vi "New Image.vi"(8 "error in (no error)":errorcluster, 9 "Buffer Number":i32, 10 "Image":T1, 11 "IMAQ Display in":refnum<class "HIJ Vision Display.lvclass">) -> (0 "error out":errorcluster, 3 "IMAQ Display out":refnum<class "HIJ Vision Display.lvclass">)   [LabVIEW 2014, in "HIJ Vision Display.lvlib" / "HIJ Vision Display.lvclass"]
uses:
  HIJ Vision Display.lvclass
  <vilib>/vision/Image Controls.llb/IMAQ Image.ctl
  HIJ Vision Display.lvclass/HIJ Vision Display.ctl
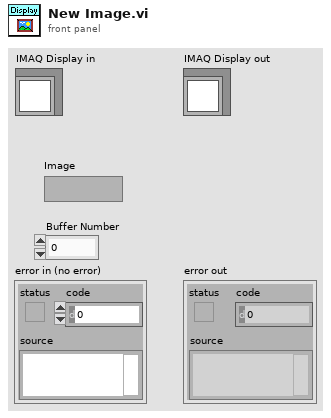
[diagram p1: front panel]
types:
  T1 = typedef "IMAQ Image.ctl" = refnum<image>
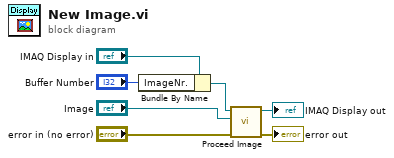
[diagram p0: block diagram]
diagram:
  n1 = Bundle By Name(cluster="IMAQ Display in", "ImageNr."="Buffer Number") -> (w2:refnum<class "HIJ Vision Display.lvclass">)
  n2 = call "Proceed Image.vi"("error in (no error)"="error in (no error)", "Image"="Image", "IMAQ Display in"=w2) -> ("error out"=→"error out":errorcluster, "HIJ Vision Display out"=→"IMAQ Display out":refnum<class "HIJ Vision Display.lvclass">)  [unwired: 7 in]
